vi "Wiimote Loop (RT RHIT's conflicted copy 2012-04-25).vi"() -> ()   [LabVIEW 2011]
doc: "This vi connects to a Wiimote via Bluetooth and passes the necessary controls to the \"Remote\" variables.\nSee Block Diagram:\n1: Open the Wiimote and acquire the device index \n2: Acquire initial calibration data\n3: Get Wiimote sensor data\n4: Set the Trigger enable condition and pass along the XY data\n5: Use a running average to smooth out the control\n6: Apply expo weight for less sensitive control and zero out dead stick offset \n7: Set XY data\n8: XY plot is data binding to network variable for the XY plot on HUD from the Remote tab\n9: Use a stop button titled \"stop?\" so that the LabVIEW script can stop the vi\n10: Close the Wiimote connection\n-Ruffin"
uses:
  Wiimote.lvlib
panel:
  in  "Expo %":i32(slide)=1 scale=0.0..100.0
  out "Analog Stick":cluster{dbl, dbl}[](graph)
  out "error out":errorcluster
  in  "stop?":bool
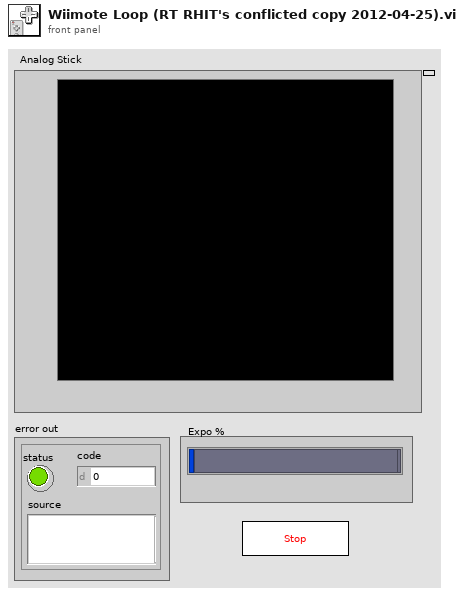
[diagram p1: front panel]
types:
  T1 = typedef "Wiimote.lvlib/Wiimote Acceleration.ctl" = cluster{"Acceleration X":dbl, "Acceleration Y":dbl, "Acceleration Z":dbl}
  T2 = cluster{"Wiimote 0G Calibration":T1, "Wiimote 1G Calibration":T1, "Nunchuk 0G Calibration":T1, "Nunchuk 1G Calibration":T1}
  T3 = typedef "Wiimote.lvlib/Wiimote Point.ctl" = cluster{"X":u16, "Y":u16}
  T4 = typedef "Wiimote.lvlib/Wiimote Buttons.ctl" = cluster{"D-Pad Left":bool, "D-Pad Right":bool, "D-Pad Down":bool, "D-Pad Up":bool, "Plus":bool, "Two":bool, "One":bool, "B":bool, "A":bool, "Minus":bool, "Home":bool}
  T5 = typedef "Wiimote.lvlib/Nunchuk Buttons.ctl" = cluster{"C":bool, "Z":bool}
  T6 = cluster{"Acceleration Calibrated Out":T1, "Acceleration Calibrated Out":T1, T3[], "Wiimote Buttons":T4, "Nunchuk Buttons":T5, "Nunchuk Analog Stick":cluster{"X":dbl, "Y":dbl}}
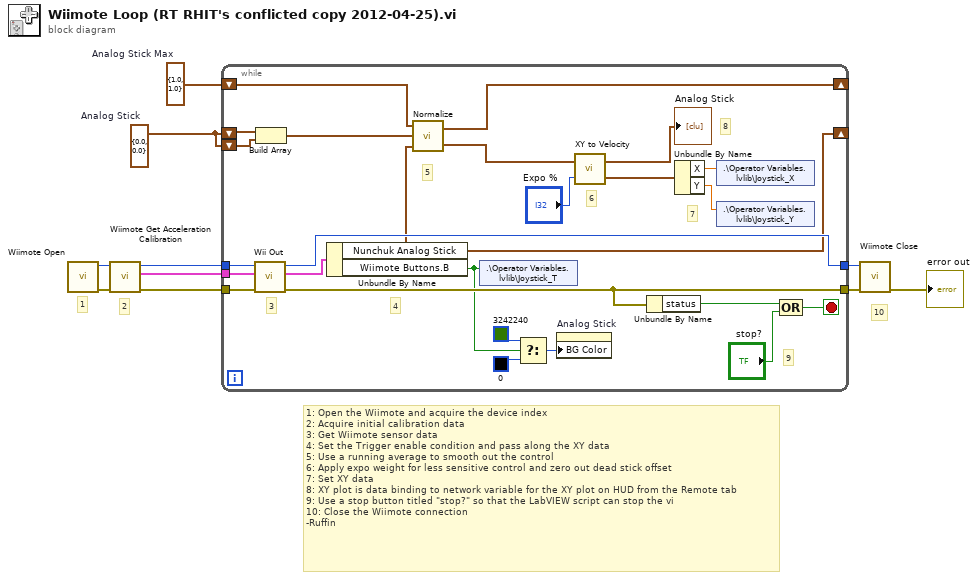
[diagram p0: block diagram]
diagram:
  w2 = cluster{"X":dbl, "Y":dbl} {"X"=1.0, "Y"=1.0}  # Analog Stick Max
  w1 = cluster{"X":dbl, "Y":dbl} {"X"=0.0, "Y"=0.0}  # Analog Stick
  # "1:\tOpen the Wiimote and acquire the device index \n2:\tAcquire initial calibration data\n3:\tGet Wiimote sensor data\n4:\tSet the Trigger enable condition and pass along the XY data\n5:\tUse a running average to smooth out the control\n6:\tApply expo weight for less sensitive control and zero out dead stick offset \n7:\tSet XY data\n8:\tXY plot is data binding to network variable for the XY plot on HUD from the Remote tab\n9:\tUse a stop button titled \"stop?\" so that the LabVIEW script can stop the vi\n10:\tClose the Wiimote connection\n-Ruffin"
  # "10"
  # "2"
  # "1"
  n1 = call "Wiimote Open.vi"() -> ("error out"=w10:errorcluster, "hWiimoteHandle"=w9:u32)  [unwired: 10 in]
  n2 = call "Wiimote Get Acceleration Calibration.vi"("error in"=w10, "hWiimoteHandle in"=w9) -> ("error out"=w8:errorcluster, "Calibration Data Out"=w7:T2, "hWiimoteHandle out"=w6:u32)  [unwired: 7 in]
  n3 = while {
    tunnel: w8 -> [w35]
    tunnel: w7 -> [w34]
    tunnel: w6 -> [w33]
    tunnel: [w32] -> w5
    tunnel: [w25] -> w3
    shift-right: [w16] -> _
    shift-left: w1 -> [w19]
    shift-right: [w20] -> _
    shift-left: w2 -> [w21]
    shift-left: w1 -> [w18]
    stop <- w28 stop-if-true
    # "9"
    # "8"
    # "7"
    # "6"
    # "5"
    # "4"
    # "3"
    n4 = call "Wii Out.vi"("error in"=w35, "Calibration Data In"=w34, "index"=w33) -> ("error out"=w25:errorcluster, "Wii output cluster"=w31:T6, "hWiimoteHandle out"=w32:u32)  [unwired: 2 in]
    n5 = Build Array(w19, w18) -> (w17:cluster{"X":dbl, "Y":dbl}[])
    n6 = Unbundle By Name(w31) -> ("Nunchuk Analog Stick"=w16:cluster{"X":dbl, "Y":dbl}, "Wiimote Buttons.B"=w11:bool)
    n7 = call "Normalize.vi"("Analog Stick"=w16, "Past Analog Stick"=w17, "Analog Stick Max"=w21) -> ("Normalized Analog Stick Out"=w15:cluster{"X":dbl, "Y":dbl}, "Analog Stick Max Out"=w20:cluster{"X":dbl, "Y":dbl})
    n8 = shared-variable ".\\Operator Variables.lvlib\\Joystick_T"(w11) -> ()  [unwired: 1 in, 1 out]
    n9 = Select(t=u32 3242240, s=w11, f=u32 0) -> (s? t:f=w12:u32)
    n10 = property on="Analog Stick" class="XYGraph (strict)"("BG Color"=w12) -> ()  [unwired: 2 in, 2 out]
    n11 = call "XY to Velocity.vi"("Expo"="Expo %", "Nunchuk Analog Stick In"=w15) -> ("X and Y"=w24:cluster{"X":dbl, "Y":dbl}, "Nunchuk Analog Stick"=→"Analog Stick":cluster{dbl, dbl}[])
    n12 = Unbundle By Name(w25) -> ("status"=w30:bool)
    n13 = Unbundle By Name(w24) -> ("X"=w23:dbl, "Y"=w22:dbl)
    n14 = shared-variable ".\\Operator Variables.lvlib\\Joystick_X"(w23) -> ()  [unwired: 1 in, 1 out]
    n15 = shared-variable ".\\Operator Variables.lvlib\\Joystick_Y"(w22) -> ()  [unwired: 1 in, 1 out]
    n16 = Compound Arithmetic op=OR(w30, "stop?") -> (w28:bool)
  }
  n17 = call "Wiimote Close.vi"("error in"=w3, "hWiimoteHandle in"=w5) -> ("error out"=→"error out":errorcluster)  [unwired: 9 in]
